vi "Initialize MeasurementLink Session.vi"(7 "remote connection options":T2, 8 "error in":errorcluster, 9 "initialize and close session behavior":T1, 10 "session initialization parameters":T3, 11 "session factory in":refnum<class "Session Factory.lvclass">) -> (0 "error out":errorcluster, 2 "session out":variant, 3 "session factory out":refnum<class "Session Factory.lvclass">)   [LabVIEW 2021, in "Session Management niSwitch.lvlib" / "Session Factory.lvclass"]
doc: "Creates a new session using the provided <b>session initialization parameters</b>. If the session represents a remote session, <b>initialize and close session behavior</b> determines whether creating the local session creates a new session on the server or attaches to an existing session on the server."
uses:
  Session Factory.lvclass
  <vilib>/Plug-In SDKs/Sessions/Instrument/ISession Factory/Session Initialization Parameters.ctl
  <vilib>/Plug-In SDKs/Sessions/Instrument/ISession Factory/Remote Connection Options.ctl
  <vilib>/Plug-In SDKs/Sessions/Instrument/ISession Factory/Initialize and Close Session Behavior.ctl
  NI Switch Client/RPC Messages/niswitch_grpc_InitWithTopologyRequest.ctl
  NI Switch Client/RPC Messages/nidevice_grpc_SessionInitializationBehavior.ctl
  Session Factory.lvclass/Session Factory.ctl
  NI Switch Client/NI Switch Client.lvlib
  <vilib>/Plug-In SDKs/Sessions/Instrument/ISession Factory/ISession Factory.lvclass
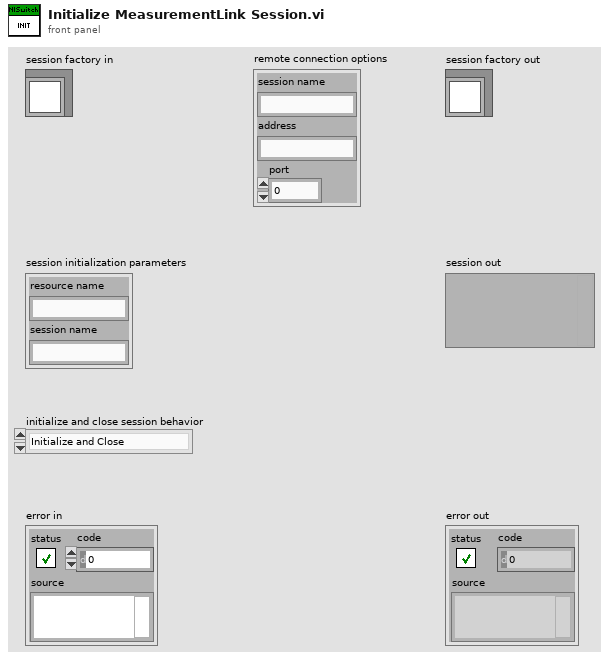
[diagram p1: front panel]
types:
  T1 = typedef "NI Session Management Instrument.lvlib/ISession Factory.lvclass/Initialize and Close Session Behavior.ctl" = enum16{"Initialize and Close", "Attach and Detach", "Initialize and Detach", "Attach and Close"}
  T2 = typedef "NI Session Management Instrument.lvlib/ISession Factory.lvclass/Remote Connection Options.ctl" = cluster{"session name":string, "address":string, "port":u32}
  T3 = typedef "NI Session Management Instrument.lvlib/ISession Factory.lvclass/Session Initialization Parameters.ctl" = cluster{"resource name":string, "session name":string}
  T4 = typedef "NI Switch Client.lvlib/niswitch_grpc_InitWithTopologyRequest.ctl" = cluster{"session_name":string, "resource_name":string, "topology":string, "simulate":bool, "reset_device":bool, "initialization_behavior":T5}
  T5 = typedef "NI Switch Client.lvlib/nidevice_grpc_SessionInitializationBehavior.ctl" = enum32{"SESSION_INITIALIZATION_BEHAVIOR_UNSPECIFIED", "SESSION_INITIALIZATION_BEHAVIOR_INITIALIZE_NEW", "SESSION_INITIALIZATION_BEHAVIOR_ATTACH_TO_EXISTING"}
  T6 = typedef "niSwitch Topologies.ctl" = string
  T7 = typedef "grpc-lvsupport-release.lvlib/grpcId.ctl" = u64
  T8 = typedef "NI Switch Client.lvlib/niswitch_grpc_InitWithTopologyResponse.ctl" = cluster{"status":i32, "vi":T9, "error_message":string, "new_session_initialized":bool}
  T9 = typedef "NI Switch Client.lvlib/nidevice_grpc_Session.ctl" = cluster{"nidevice_grpc_Session_session":refnum<class "nidevice_grpc_Session_session.lvclass">}
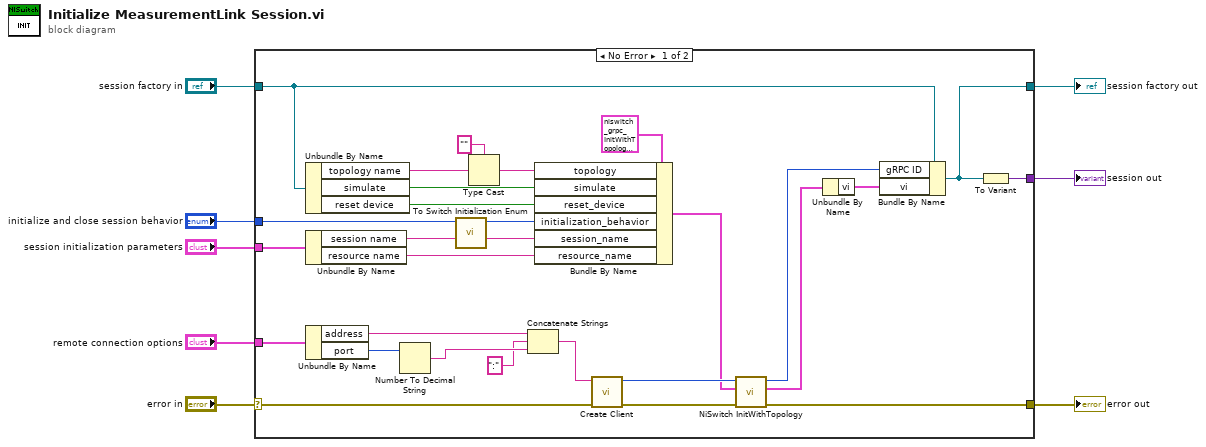
[diagram p0: block diagram]
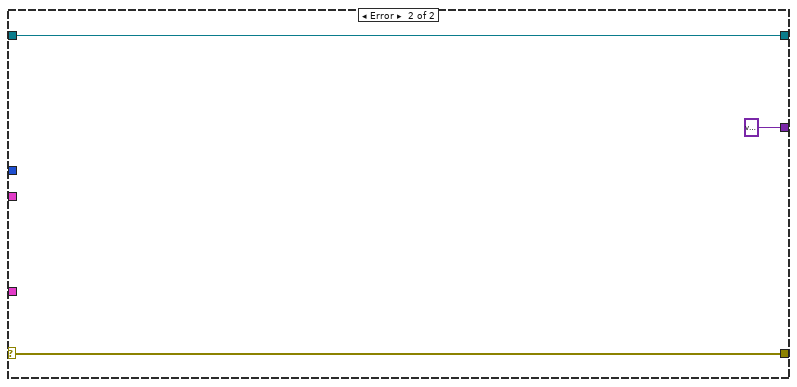
[diagram p2: hidden frame]
diagram:
  n1 = case shown="No Error" "error in" {
    selector: "error in" -> [w35 w39]
    tunnel: [w34 w39] -> w5
    tunnel: "session initialization parameters" -> [w33 _]
    tunnel: [w9 w38] -> w6
    tunnel: "session factory in" -> [w10 w38]
    tunnel: "initialize and close session behavior" -> [w29 _]
    tunnel: "remote connection options" -> [w20 _]
    tunnel: [w11 variant ("Variant")] -> w1
    frame No Error {
      n2 = Unbundle By Name(w10) -> ("topology name"=w24:T6, "simulate"=w27:bool, "reset device"=w26:bool)
      n3 = Unbundle By Name(w33) -> ("session name"=w32:string, "resource name"=w31:string)
      n4 = Unbundle By Name(w20) -> ("address"=w12:string, "port"=w19:u32)
      n5 = Number To Decimal String(number=w19) -> (decimal integer string=w18:string)  [unwired: 1 in]
      n6 = call "To Switch Initialization Enum.vi"("initialize and close session behavior"=w29) -> ("initialization_behavior"=w28:T5)  [unwired: 10 in]
      n7 = Type Cast(type="" ("topology"), x=w24) -> (*(type *) &x=w23:string)
      n8 = Concatenate Strings(w12, ":" ("string"), w18) -> (w30:string)
      n9 = Bundle By Name(cluster=T4 {"session_name"="", "resource_name"="", "topology"="", "simulate"=FALSE, "reset_device"=FALSE, "initialization_behavior"=enum."SESSION_INITIALIZATION_BEHAVIOR_UNSPECIFIED"} ("Request Data"), "topology"=w23, "simulate"=w27, "reset_device"=w26, "initialization_behavior"=w28, "session_name"=w32, "resource_name"=w31) -> (w21:T4)
      n10 = call "Create Client.vi"("error in"=w35, "address"=w30) -> ("error out"=w36:errorcluster, "gRPC ID Out"=w22:T7)  [unwired: 8 in]
      n11 = call "NiSwitch InitWithTopology.vi"("error in"=w36, "Request Data"=w21, "gRPC ID"=w22) -> ("error out"=w34:errorcluster, "Response Data"=w14:T8, "gRPC ID out"=w15:T7)  [unwired: 6 in]
      n12 = Unbundle By Name(w14) -> ("vi"=w13:T9)
      n13 = Bundle By Name(cluster=w10, "gRPC ID"=w15, "vi"=w13) -> (w9:refnum<class "Session Factory.lvclass">)
      n14 = To Variant(anything=w9) -> (Variant=w11:variant)
    }
    frame Error {
    }
  }
  "error out" <- w5
  "session factory out" <- w6
  "session out" <- w1
